vi "Template Server Example.vi"() -> ()   [LabVIEW 2019, in "Template Server.lvlib"]
uses:
  Template Server.lvlib
  Class/Template Server.lvclass/Template Server.ctl
  Class/Template Server.lvclass
panel:
  in  "Enable Async Mode":bool
  out "error out":errorcluster
  in  "Stop":bool
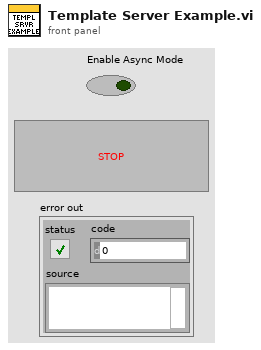
[diagram p1: front panel]
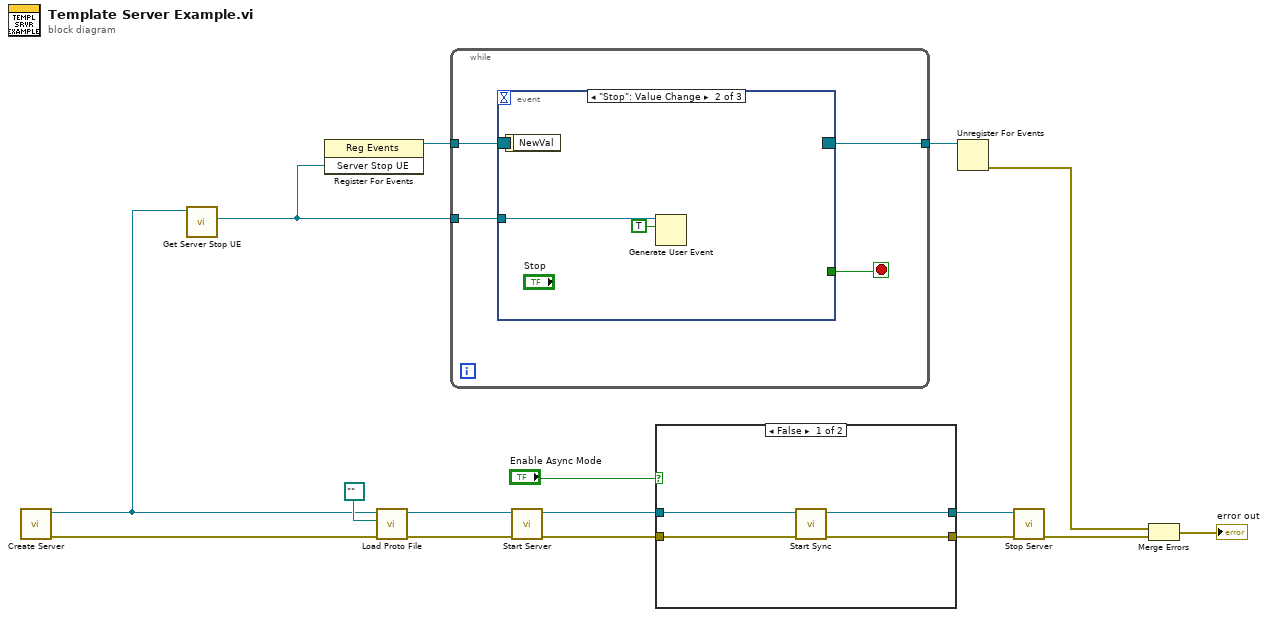
[diagram p0: block diagram]
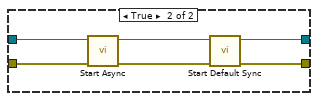
[diagram p2: hidden frame]
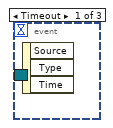
[diagram p3: hidden frame]
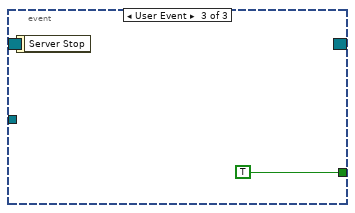
[diagram p4: hidden frame]
diagram:
  n1 = call "Create Server.vi"() -> ("error out"=w16:errorcluster, "OOP Server out"=w12:refnum<class "Template Server.lvclass">)  [unwired: 10 in]
  n2 = call "Get Server Stop UE.vi"("OOP Server in"=w12) -> ("Server Stop UE"=w10:refnum<user-event>)  [unwired: 9 in, 1 out]
  n3 = register-events(w10) -> (reference out=w11:refnum<event-registration>)  [unwired: 2 in, 1 out]
  n4 = call "Load Proto File.vi"("error in (no error)"=w16, "Proto File Path"=path "", "OOP Server in"=w12) -> ("error out"=w5:errorcluster, "OOP Server out"=w4:refnum<class "Template Server.lvclass">)  [unwired: 7 in]
  n5 = while {
    tunnel: w10 -> [w20]
    tunnel: w11 -> [w19]
    tunnel: [w17] -> w9
    stop <- w18 stop-if-true
    n6 = event shown="[1] \"Stop\": Value Change" {
      selector: w19 -> [_ _ _]
      dyn-events: [_ _ _] -> w17
      timeout: _ -> [_ _ _]
      tunnel: w20 -> [_ w22 _]
      tunnel: [_ _ TRUE] -> w18
      event Timeout {
        n7 = event-data() -> ()  [unwired: 1 in, 3 out]
      }
      event "Stop": Value Change {
        n8 = event-data() -> ()  [unwired: 1 in, 1 out]
        n9 = Generate User Event(user event=w22, event data cluster=TRUE ("event data")) -> ()  [unwired: 2 in, 2 out]
      }
      event User Event {
        n10 = event-data() -> ()  [unwired: 1 in, 1 out]
      }
    }
  }
  n11 = call "Start Server.vi"("error in (no error)"=w5, "OOP Server in"=w4) -> ("error out"=w3:errorcluster, "OOP Server out"=w2:refnum<class "Template Server.lvclass">)  [unwired: 8 in]
  n12 = case shown="False" "Enable Async Mode" {
    tunnel: [w24 w33] -> w15
    tunnel: [w25 w32] -> w14
    tunnel: w3 -> [w27 w31]
    tunnel: w2 -> [w26 w30]
    frame False {
      n13 = call "Start Sync.vi"("error in (no error)"=w27, "OOP Server in"=w26) -> ("error out"=w24:errorcluster, "OOP Server out"=w25:refnum<class "Template Server.lvclass">)  [unwired: 8 in]
    }
    frame True {
      n14 = call "Start Async.vi"("error in (no error)"=w31, "OOP Server in"=w30) -> ("error out"=w29:errorcluster, "OOP Server out"=w28:refnum<class "Template Server.lvclass">)  [unwired: 8 in]
      n15 = call "Start Default Sync.vi"("error in (no error)"=w29, "OOP Server in"=w28) -> ("error out"=w33:errorcluster, "OOP Server out"=w32:refnum<class "Template Server.lvclass">)  [unwired: 8 in]
    }
  }
  n16 = Unregister For Events(event registration refnum=w9) -> (error out=w7:errorcluster)  [unwired: 1 in]
  n17 = call "Stop Server.vi"("error in (no error)"=w15, "OOP Server in"=w14) -> ("error out"=w8:errorcluster)  [unwired: 8 in, 1 out]
  n18 = Merge Errors(w7, w8) -> (→"error out":errorcluster)
